vi "Hermite Path.vi"(0 "Initial":T5, 1 "s_max (1)":dbl=1.0, 5 "Final":T4, 7 "backwards":bool, 9 "array_len":u32, 12 "s_min (0)":dbl) -> (4 "Output":T6)   [LabVIEW 2019]
doc: "__declspec(dllexport) void __stdcall HermitePath(double initial_x, double initial_y, double initial_theta,\n double final_x, double final_y, double final_theta,\n double initial_velocity, double final_velocity, unsigned char backwards,\n double extra_distance_initial, double extra_distance_final,\n double initial_angular_velocity, double final_angular_velocity,\n double s_min, double s_max, unsigned int array_len,\n double* path_x, double* path_y, double* path_theta);"
uses:
  Typedef/Trajectory.ctl
  Geometry/Typedef/Pose2d.ctl
  Geometry/Typedef/Translation2d.ctl
  Geometry/Typedef/Rotation2d.ctl
  main.dll
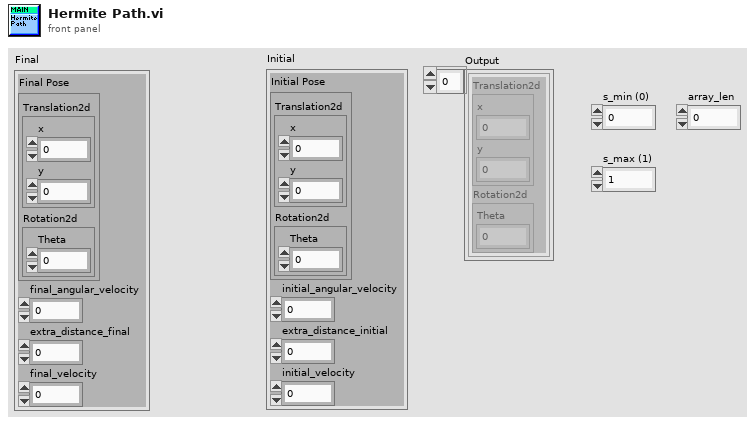
[diagram p1: front panel]
types:
  T1 = typedef "Pose2d.ctl" = cluster{"Translation2d":T2, "Rotation2d":T3}
  T2 = typedef "Translation2d.ctl" = cluster{"x":dbl, "y":dbl}
  T3 = typedef "Rotation2d.ctl" = cluster{"Theta":dbl}
  T4 = cluster{"Final Pose":T1, "final_angular_velocity":dbl, "extra_distance_final":dbl, "final_velocity":dbl}
  T5 = cluster{"Initial Pose":T1, "initial_angular_velocity":dbl, "extra_distance_initial":dbl, "initial_velocity":dbl}
  T6 = typedef "Trajectory.ctl" = T1[]
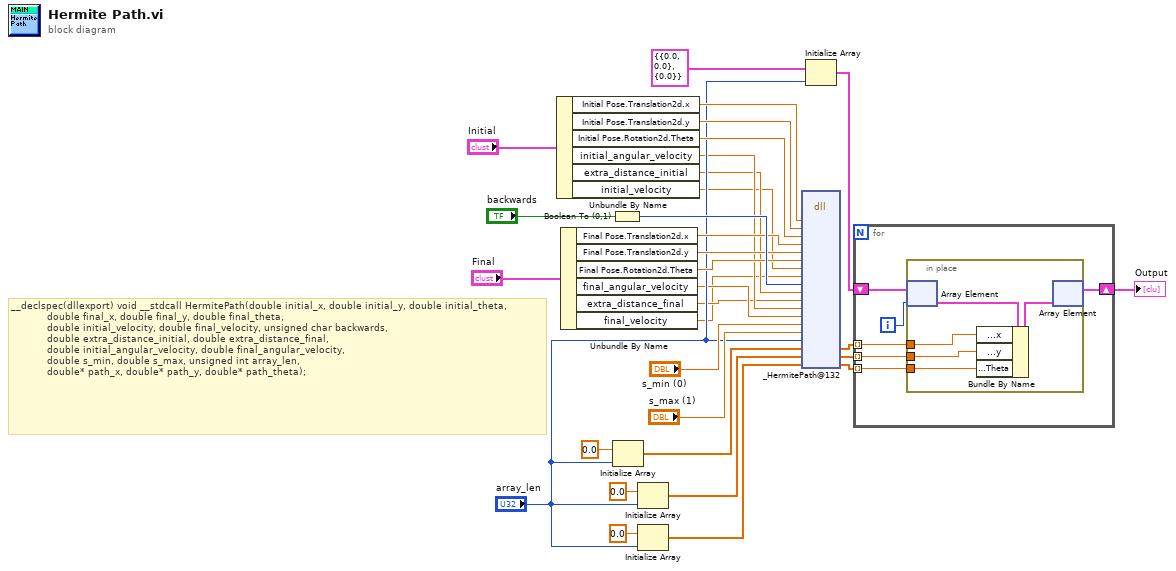
[diagram p0: block diagram]
diagram:
  # "__declspec(dllexport) void __stdcall HermitePath(double initial_x, double initial_y, double initial_theta,\n            double final_x, double final_y, double final_theta,\n            double initial_velocity, double final_velocity, unsigned char backwards,\n            double extra_distance_initial, double extra_distance_final,\n            double initial_angular_velocity, double final_angular_velocity,\n            double s_min, double s_max, unsigned int array_len,\n            double* path_x, double* path_y, double* path_theta);"
  n1 = Unbundle By Name("Initial") -> ("Initial Pose.Translation2d.x"=w21:dbl, "Initial Pose.Translation2d.y"=w20:dbl, "Initial Pose.Rotation2d.Theta"=w19:dbl, "initial_angular_velocity"=w7:dbl, "extra_distance_initial"=w6:dbl, "initial_velocity"=w4:dbl)
  n2 = Unbundle By Name("Final") -> ("Final Pose.Translation2d.x"=w18:dbl, "Final Pose.Translation2d.y"=w17:dbl, "Final Pose.Rotation2d.Theta"=w16:dbl, "final_angular_velocity"=w3:dbl, "extra_distance_final"=w2:dbl, "final_velocity"=w1:dbl)
  n3 = Boolean To (0,1)(Boolean="backwards") -> (0, 1=w30:i16)
  n4 = Initialize Array(0.0 ("element"), "array_len") -> (w27:dbl[])
  n5 = Initialize Array(0.0 ("element"), "array_len") -> (w25:dbl[])
  n6 = Initialize Array(0.0 ("element"), "array_len") -> (w23:dbl[])
  n7 = dll-call lib="C:/Users/Will/Src/Robotics-Toolkit/Trajectory/Quintic Hermite/main.*" fn="_HermitePath@132"("initial_x"=w21, "initial_y"=w20, "initial_theta"=w19, "final_x"=w18, "final_y"=w17, "final_theta"=w16, "initial_velocity"=w4, "final_velocity"=w1, "backwards"=w30, "extra_distance_initial"=w6, "extra_distance_final"=w2, "initial_angular_velocity"=w7, "final_angular_velocity"=w3, "s_min"="s_min (0)", "s_max"="s_max (1)", "array_len"="array_len", "path_x"=w27, "path_y"=w25, "path_theta"=w23) -> ("path_x"=w13:dbl[], "path_y"=w12:dbl[], "path_theta"=w11:dbl[])  [unwired: 20 in, 2 out]
  n8 = Initialize Array(T1 {"Translation2d"={"x"=0.0, "y"=0.0}, "Rotation2d"={"Theta"=0.0}} ("Final Pose 2"), "array_len") -> (w10:T1[])
  n9 = for {
    tunnel: w13 -> [w35] mode=indexing
    tunnel: w12 -> [w34] mode=indexing
    tunnel: w11 -> [w33] mode=indexing
    shift-right: [w32] -> w9
    shift-left: w10 -> [w36]
    i -> [w37]
    n10 = in-place {
      in-place-border: w35 -> [w41]
      in-place-border: w34 -> [w40]
      in-place-border: w33 -> [w39]
      n11 = in-place-array #1(w36, w37) -> (w42:T1)
      n12 = Bundle By Name(cluster=w42, "Translation2d.x"=w41, "Translation2d.y"=w40, "Rotation2d.Theta"=w39) -> (w38:T1)
      n13 = in-place-array #1(w38) -> (w32:T1[])  [unwired: 1 out]
    }
  }
  "Output" <- w9
